vi "Multiple VIs in a Subpanel.vi"() -> ()   [LabVIEW 2023]
doc: "This example shows how to view VIs in a Subpanel control."
panel:
  in  "VI to Display":u16(ring) items=["Sine Graph", "Random Data Chart", "Current Time"]
  in  "Stop":bool
  # "Overview: Demonstrates the use of the Subpanel control to display different VI panels.\nInstructions:\n1. Run the VI.\n2. Select different options in the VI to Display ring to display different VIs in the subpanel.\n3. Click Stop to stop the VI."
  # "The VI Properties of the inserted VI govern its appearance in the Subpanel control. For example, all of the plugin VIs for this example have their scrollbars disabled. Thus, scrollbars do not appear within the Subpanel control."
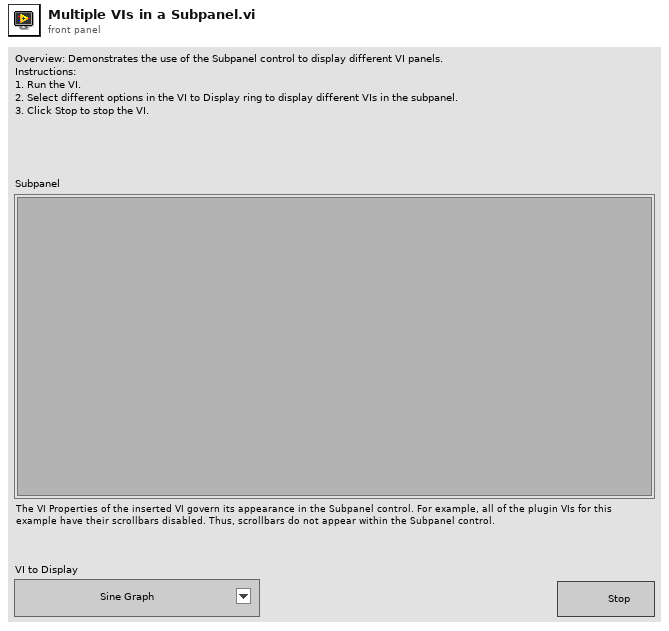
[diagram p1: front panel]
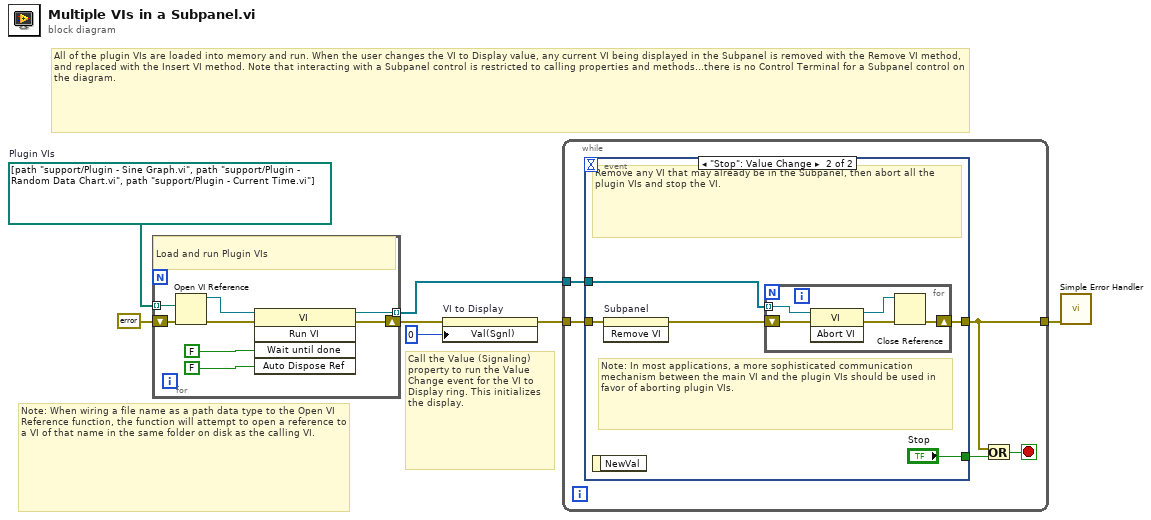
[diagram p0: block diagram]
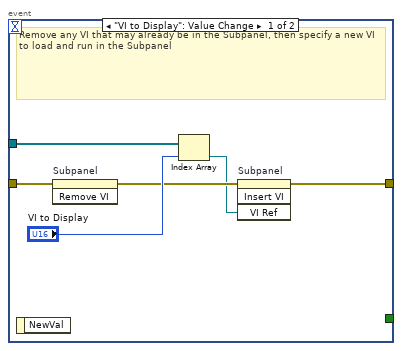
[diagram p2: hidden frame]
diagram:
  w4 = path[] [path "support/Plugin - Sine Graph.vi", path "support/Plugin - Random Data Chart.vi", path "support/Plugin - Current Time.vi"]  # Plugin VIs
  # "All of the plugin VIs are loaded into memory and run. When the user changes the VI to Display value, any current VI being displayed in the Subpanel is removed with the Remove VI method, and replaced with the Insert VI method. Note that interacting with a Subpanel control is restricted to calling properties and methods...there is no Control Terminal for a Subpanel control on the diagram."
  # "Note: When wiring a file name as a path data type to the Open VI Reference function, the function will attempt to open a reference to a VI of that name in the same folder on disk as the calling VI."
  # "Call the Value (Signaling) property to run the Value Change event for the VI to Display ring. This initializes the display."
  n1 = for {
    tunnel: w4 -> [w11] mode=indexing
    tunnel: [w10] -> w1 mode=indexing
    shift-right: [w8] -> w2
    shift-left: errorcluster {"status"=FALSE, "code"=0, "source"=""} ("error constant") -> [w9]
    # "Load and run Plugin VIs"
    n2 = Open VI Reference(vi path=w11, error in (no error)=w9) -> (vi reference=w12:refnum<vi>, error out=w13:errorcluster)  [unwired: 4 in]
    n3 = invoke class="VI" method="Run VI"(reference=w12, error in=w13, "Wait until done"=FALSE ("Wait Until Done"), "Auto Dispose Ref"=FALSE ("Auto Dispose Reference")) -> (reference out=w10:refnum<vi>, error out=w8:errorcluster)  [unwired: 1 in, 3 out]
  }
  n4 = property on="VI to Display" class="Ring (strict)"(error in=w2, "Val(Sgnl)"=u16 0 ("Value (Signaling)")) -> (error out=w7:errorcluster)  [unwired: 1 in, 1 out]
  n5 = while {
    tunnel: w7 -> [w16]
    tunnel: [w18] -> w5
    tunnel: w1 -> [w17]
    stop <- w19 stop-if-true
    n6 = event shown="[1] \"Stop\": Value Change" {
      selector: _ -> [_ _]
      dyn-events: _ -> [_ _]
      timeout: _ -> [_ _]
      tunnel: [_ "Stop"] -> w20
      tunnel: [w25 w28] -> w18
      tunnel: w17 -> [w24 w29]
      tunnel: w16 -> [w21 w27]
      event "VI to Display": Value Change {
        # "Remove any VI that may already be in the Subpanel, then specify a new VI to load and run in the Subpanel"
        n7 = event-data() -> ()  [unwired: 1 in, 1 out]
        n8 = invoke on="Subpanel" class="SubPnl" method="Remove VI"(error in=w21) -> (error out=w23:errorcluster)  [unwired: 2 in, 2 out]
        n9 = Index Array(array=w24, index="VI to Display") -> (element=w22:refnum<vi>)
        n10 = invoke on="Subpanel" class="SubPanel" method="Insert VI"(error in=w23, "VI Ref"=w22) -> (error out=w25:errorcluster)  [unwired: 2 in, 3 out]
      }
      event "Stop": Value Change {
        # "Note: In most applications, a more sophisticated communication mechanism between the main VI and the plugin VIs should be used in favor of aborting plugin VIs."
        # "Remove any VI that may already be in the Subpanel, then abort all the plugin VIs and stop the VI."
        n11 = event-data() -> ()  [unwired: 1 in, 1 out]
        n12 = invoke on="Subpanel" class="SubPnl" method="Remove VI"(error in=w27) -> (error out=w30:errorcluster)  [unwired: 2 in, 2 out]
        n13 = for {
          shift-right: [w32] -> w28
          shift-left: w30 -> [w36]
          tunnel: w29 -> [w35] mode=indexing
          n14 = invoke class="VI" method="Abort VI"(reference=w35, error in=w36) -> (reference out=w33:refnum<vi>, error out=w34:errorcluster)  [unwired: 1 in, 1 out]
          n15 = Close Reference(reference=w33, error in (no error)=w34) -> (error out=w32:errorcluster)
        }
      }
    }
    n16 = Or(x=w18, y=w20) -> (x .or. y?=w19:bool)
  }
  n17 = call <vilib>:"Simple Error Handler.vi"("error in (no error)"=w5) -> ()  [unwired: 4 in, 5 out]
